vi "Update Channel Settings (Array).vi"(2 "Channel Settings ducktype":T4(array[cluster]), 3 "Channel Settings in":T1[](array[typedef])) -> (0 "Channel Settings out":T1[](array[typedef]))   [LabVIEW 2021, in "Settings.lvlib"]
uses:
  Acquisition/IO Device.ctl
  Acquisition/Sensor Type.ctl
  Acquisition/Channel Settings.ctl
  Settings.lvlib
  Acquisition/Acquisition.lvlib
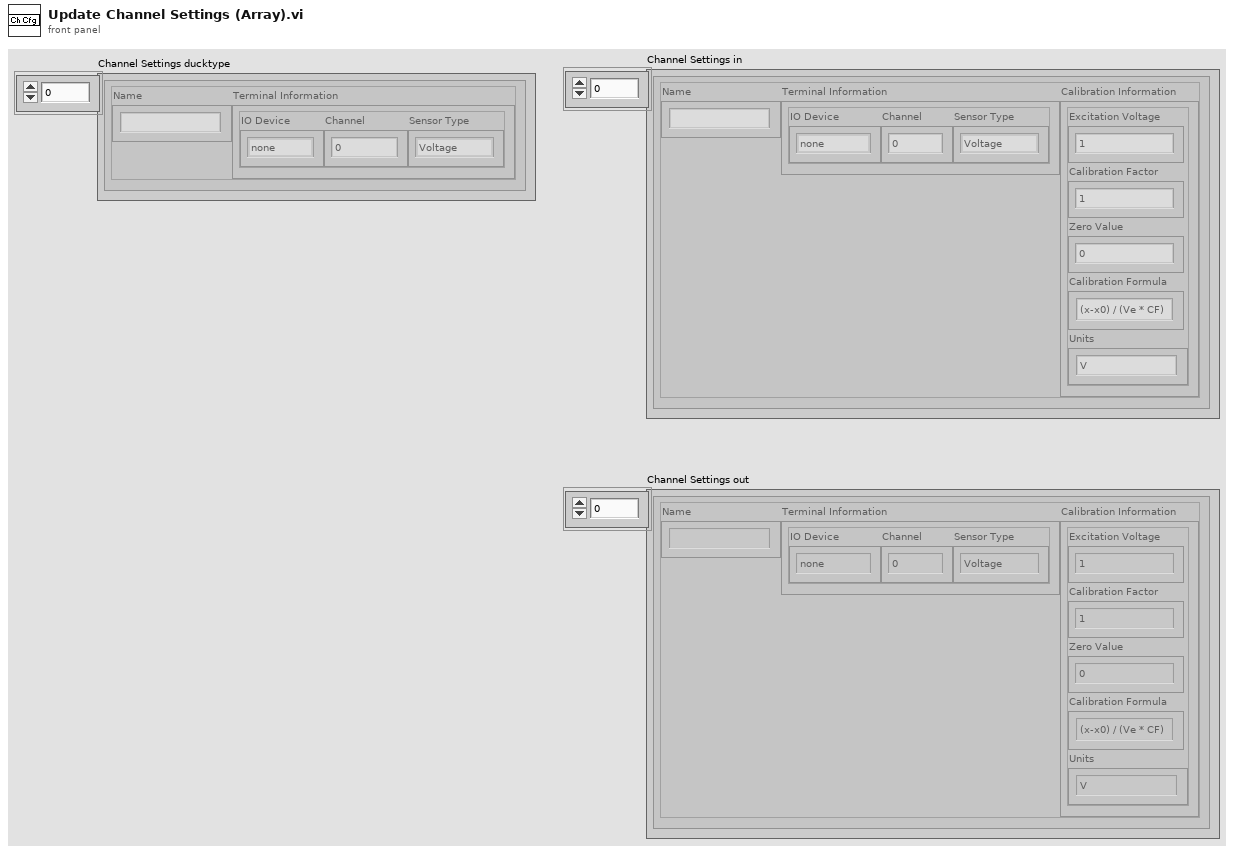
[diagram p1: front panel]
types:
  T1 = typedef "Acquisition.lvlib/Channel Settings.ctl" = cluster{"Name":string, "Terminal Information":cluster{"IO Device":T2, "Channel":i32, "Sensor Type":T3}, "Calibration Information":cluster{"Excitation Voltage":dbl, "Calibration Factor":dbl, "Zero Value":dbl, "Calibration Formula":string, "Units":string}}
  T2 = typedef "Acquisition.lvlib/IO Device.ctl" = enum16{"none", "9219", "9401"}
  T3 = typedef "Acquisition.lvlib/Sensor Type.ctl" = enum16{"Voltage", "Load", "Pressure", "Encoder"}
  T4 = cluster{"Name":string, "Terminal Information":cluster{"IO Device":T2, "Channel":i32, "Sensor Type":T3}}[]
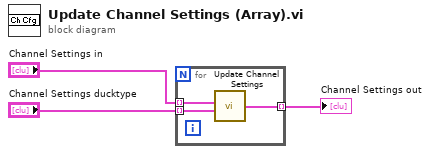
[diagram p0: block diagram]
diagram:
  n1 = for {
    tunnel: "Channel Settings in" -> [w6] mode=indexing
    tunnel: "Channel Settings ducktype" -> [w5] mode=indexing
    tunnel: [w4] -> w1 mode=indexing
    n2 = call "Update Channel Settings.vi"("Channel Settings ducktype"=w5, "Channel Settings in"=w6) -> ("Channel Settings out"=w4:T1)  [unwired: 2 in]
  }
  "Channel Settings out" <- w1
